vi "ArmGlobal.vi"() -> ()   [LabVIEW 2023]
doc: "Global varables for Arm"
uses:
  ArmPositionPreset.ctl
  ArmGamePiecePreset.ctl
panel:
  in  "Game Piece":T1
  in  "Position":T2=enum."Middle"
  out "HeadingToTarget":bool
  out "Override":bool
  out "TargetGamePiece":string
  out "TargetArmPosition":string
  out "RLEOnTarget":bool
  out "LiftOnTarget":bool
  out "ExtendOnTarget":bool
  out "ExtendPostion":dbl
  out "LiftPostion":dbl
  out "ExtendMotorOutput":dbl
  out "LiftMotorOutput":dbl
  out "ExtendPositonDemand(in)":dbl
  out "LiftPositionDemand(d)":dbl
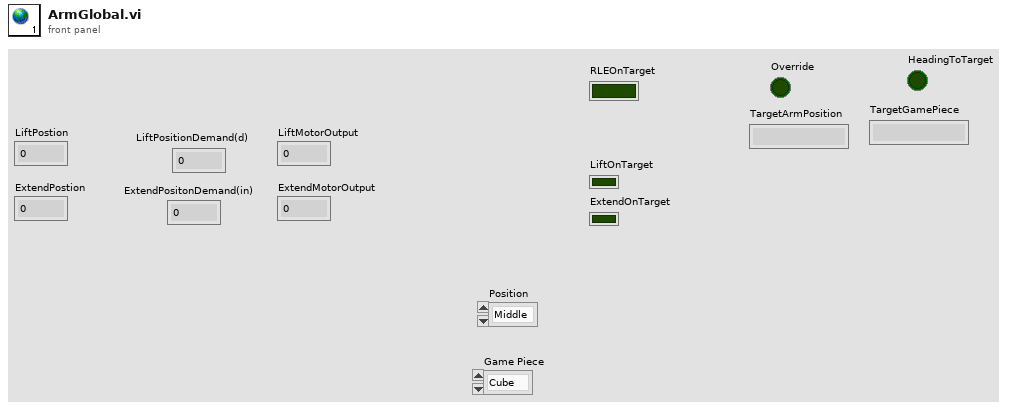
[diagram p1: front panel]
types:
  T1 = typedef "ArmGamePiecePreset.ctl" = enum16{"Cube", "Cone"}
  T2 = typedef "ArmPositionPreset.ctl" = enum16{"Upper", "Lower", "Middle", "Home", "Shelf", "Floor", "HalfFloor", "HalfHome"}
diagram:
